vi "FPGA_Twosetup.vi"() -> ()   [LabVIEW 2015]
uses:
  <vilib>/rvi/Emulation/niFpgaGetClockAttributes.vi
  <vilib>/rvi/Emulation/niFpgaSctlEmulationGetInTimedLoop.vi
  <vilib>/rvi/Emulation/niFpgaEmulationReportErrorSimple.vi
  <vilib>/rvi/eio/common/nirviEmuTemplateMethod_errors.vi
  <vilib>/rvi/interface/RandomDataEmulation/niFpgaRandomDataHandleErrors.vi
  <vilib>/rvi/Emulation/niFpgaCriticalErrorInLSC.vi
  <vilib>/eio/EIONode/EIONode.xnode
  <vilib>/rvi/DataTransferAndStorage/Container/XNode/niFpgaContainer.xnode
  <vilib>/rvi/interface/RandomDataEmulation/nirviRandomDataFpgaReadWriteTemplate.vi
panel:
  in  "stop LED illumination 2":bool
  in  "Low Period (ticks) 2":u32=40000000
  in  "High Period (ticks) 2":u32=40000000
  in  "Apply 2":bool
  in  "Output Enable 2":bool
  in  "FPGA Stop 2":bool
  in  "Half-clock time 2":u32=10
  out "ConnectorA/DIO0 2":bool=TRUE
  out "Frame Count 2":i16=5
  in  "IRQ Bit (0-31) 2":u8
  in  "Wait Until IRQ Cleared? 2":bool
  out "Timed Out? 2":bool
  out "ConnectorA/AI0 2":u16=44020
  out "ConnectorA/DIO1 2":bool
  in  "double number of samples to take per frame 2":u16=1540
  in  "Half-clocks between frames 2":u16=1600
  in  "ConnectorA/AO0 2":u16
  in  "stop LED illumination":bool
  in  "Low Period (ticks)":u32=40000000
  in  "High Period (ticks)":u32=40000000
  in  "Apply":bool
  in  "Output Enable":bool
  in  "FPGA Stop":bool
  in  "Half-clock time":u32=10
  out "ConnectorB/DIO0":bool=TRUE
  out "Frame Count":i16=5
  in  "IRQ Bit (0-31)":u8
  in  "Wait Until IRQ Cleared?":bool
  out "Timed Out?":bool
  out "ConnectorB/AI0":u16=44020
  out "ConnectorB/DIO1":bool
  in  "double number of samples to take per frame":u16=1540
  in  "Half-clocks between frames":u16=1600
  in  "ConnectorB/AO0":u16
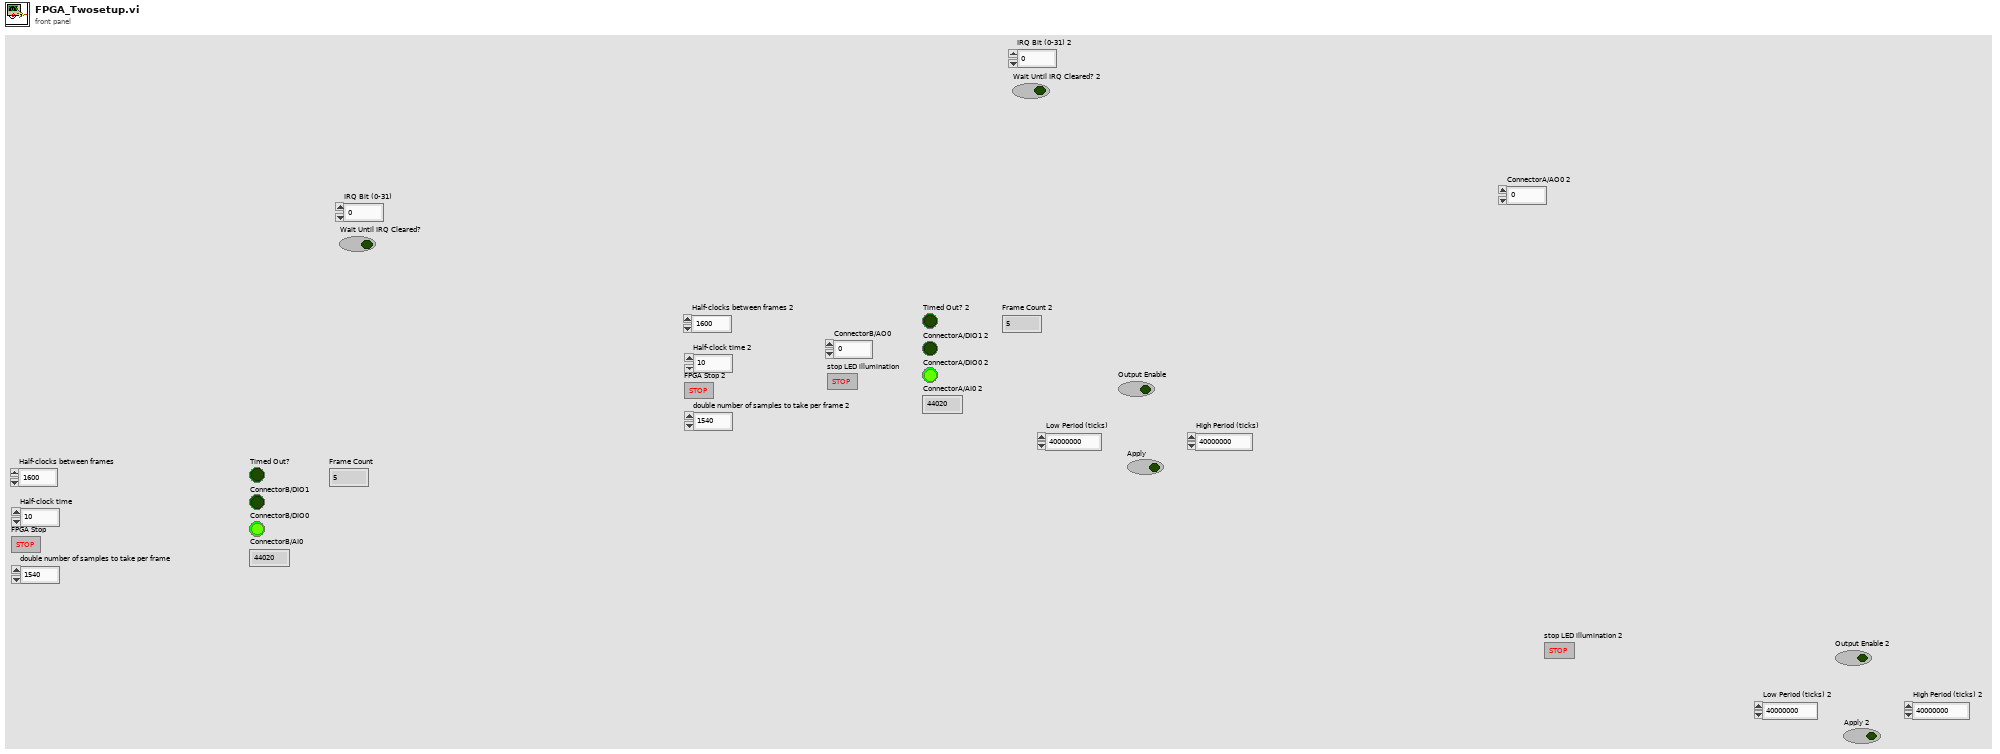
[diagram p1: front panel]
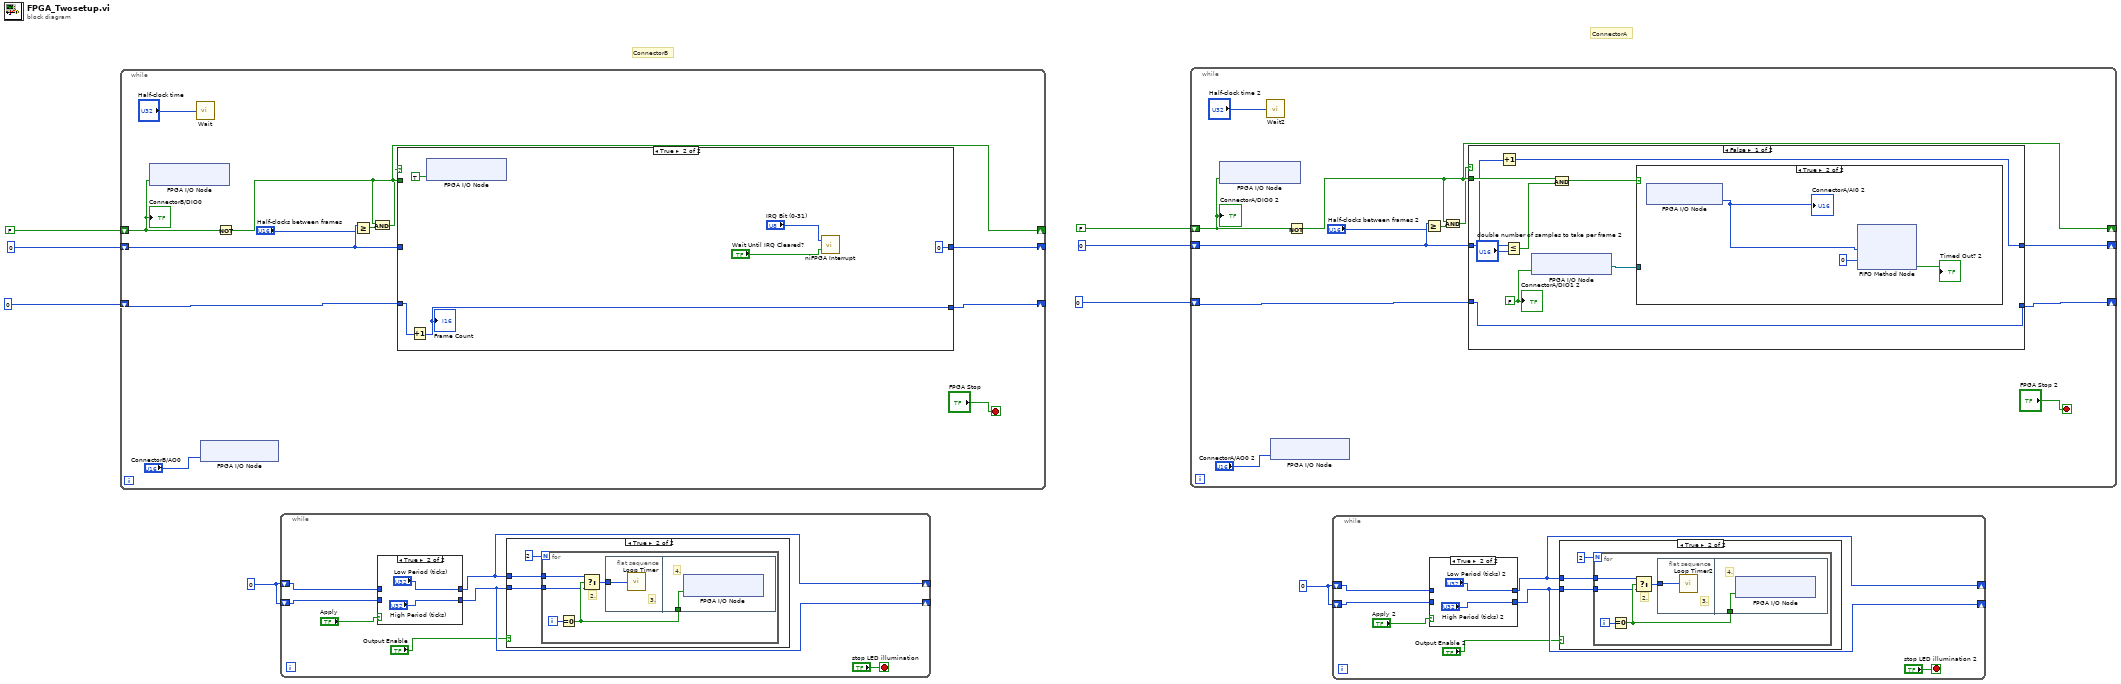
[diagram p0: block diagram]
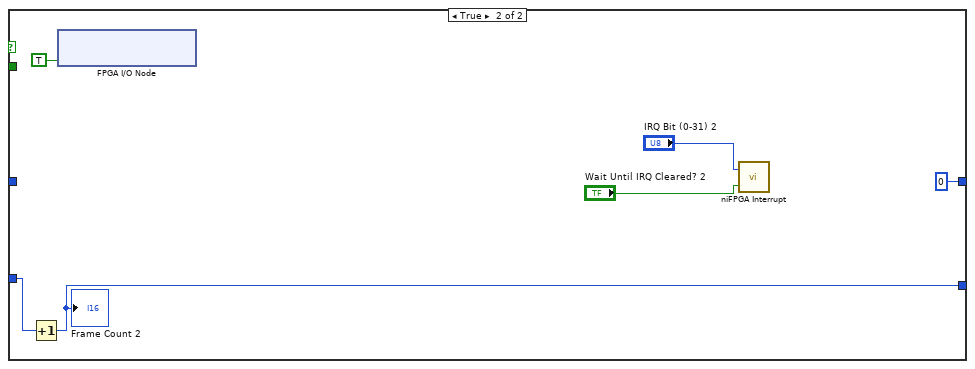
[diagram p5: hidden frame]
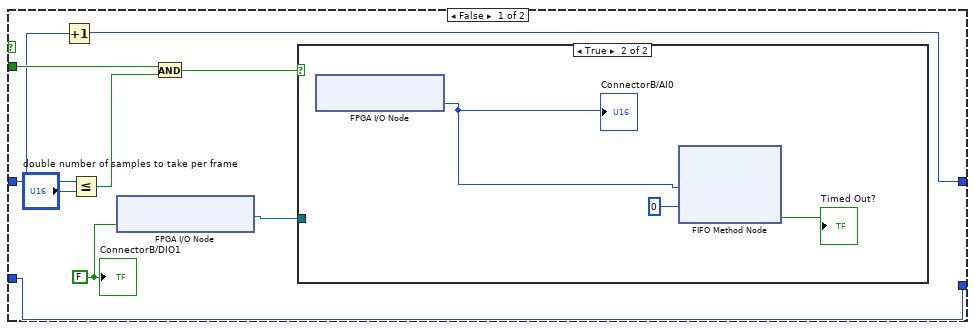
[diagram p8: hidden frame]
diagram:
  w1 = u32 0 ("High Period")
  w5 = u32 0 ("High Period")
  # "ConnectorA"
  # "ConnectorB"
  n1 = while {
    shift-right: [w19] -> _
    shift-left: FALSE ("ConnectorB/DIO0") -> [w20]
    shift-right: [w16] -> _
    shift-left: u16 0 -> [w18]
    shift-right: [w14] -> _
    shift-left: i16 0 -> [w15]
    stop <- "FPGA Stop" stop-if-true
    n2 = xnode "FPGA I/O Node"("ConnectorB/DIO0"=w20) -> ()  [unwired: 1 in, 1 out]
    n3 = call "Wait"("Count(uSec)"="Half-clock time") -> ()  [unwired: 1 out]
    n4 = xnode "FPGA I/O Node"("ConnectorB/AO0"="ConnectorB/AO0") -> ()  [unwired: 1 in, 1 out]
    n5 = Not(x=w20) -> (.not. x?=w19:bool)
    n6 = Greater Or Equal?(x=w18, y="Half-clocks between frames") -> (x >= y?=w12:bool)
    n7 = And(x=w19, y=w12) -> (x .and. y?=w10:bool)
    n8 = case shown="True" w10 {
      tunnel: w18 -> [w24 _]
      tunnel: [w22 u16 0] -> w16
      tunnel: w19 -> [w28 _]
      tunnel: w15 -> [w23 w36]
      tunnel: [w23 w35] -> w14
      frame False {
        w29 = FALSE ("ConnectorB/DIO1")
        n9 = Increment(x=w24) -> (x+1=w22:u16)
        n10 = Less Or Equal?(x=w24, y="double number of samples to take per frame") -> (x <= y?=w26:bool)
        n11 = xnode "FPGA I/O Node"("ConnectorB/DIO1"=w29) -> ("FPGA I/O Out"=w25:refnum<k21>)  [unwired: 1 in]
        n12 = And(x=w28, y=w26) -> (x .and. y?=w27:bool)
        n13 = case shown="True" w27 {
          tunnel: w25 -> [_ _]
          frame False {
          }
          frame True {
            n14 = xnode "FPGA I/O Node"() -> ("ConnectorB/AI0"=w32:u16)  [unwired: 1 in, 1 out]
            "ConnectorB/AI0" <- w32
            n15 = xnode ("FIFO Method Node")("Element"=w32, "Timeout"=0) -> ("Timed Out?"=→"Timed Out?":bool)  [unwired: 1 in, 1 out]
          }
        }
        "ConnectorB/DIO1" <- w29
      }
      frame True {
        n16 = Increment(x=w36) -> (x+1=w35:i16)
        "Frame Count" <- w35
        n17 = xnode "FPGA I/O Node"("ConnectorB/DIO1"=TRUE) -> ()  [unwired: 1 in, 1 out]
        n18 = call <vilib>:"niFPGA Interrupt.vi"("Wait Until Cleared (F)"="Wait Until IRQ Cleared?", "IRQ Number (0)"="IRQ Bit (0-31)") -> ()  [unwired: 1 in]
      }
    }
    "ConnectorB/DIO0" <- w20
  }
  n19 = while {
    shift-right: [w40] -> _
    shift-left: w5 -> [w44]
    shift-right: [w41] -> _
    shift-left: w5 -> [w43]
    stop <- "stop LED illumination" stop-if-true
    n20 = case shown="True" "Apply" {
      tunnel: [w57 "Low Period (ticks)"] -> w40
      tunnel: [w56 "High Period (ticks)"] -> w41
      tunnel: w44 -> [w57 _]
      tunnel: w43 -> [w56 _]
      frame False {
      }
      frame True {
      }
    }
    n21 = case shown="True" "Output Enable" {
      tunnel: w40 -> [_ w47]
      tunnel: w41 -> [_ w46]
      frame False {
      }
      frame True {
        n22 = for {
          N: 2 -> [_]
          tunnel: w47 -> [w50]
          tunnel: w46 -> [w49]
          i -> [w52]
          # "2."
          n23 = Equal To 0?(x=w52) -> (x = 0?=w51:bool)
          n24 = Select(t=w50, s=w51, f=w49) -> (s? t:f=w53:u32)
          n25 = flat-sequence {
            tunnel: w53 -> [w54]
            tunnel: w51 -> [w55]
            frame #0 {
              # "3."
              n26 = call "Loop Timer"("Count(Ticks)"=w54) -> ()  [unwired: 1 out]
            }
            frame #1 {
              # "4."
              n27 = xnode "FPGA I/O Node"("ConnectorB/DIO8"=w55) -> ()  [unwired: 1 in, 1 out]
            }
          }
        }
      }
    }
  }
  n28 = while {
    shift-right: [w70] -> _
    shift-left: FALSE ("ConnectorB/DIO0") -> [w71]
    shift-right: [w67] -> _
    shift-left: u16 0 -> [w69]
    shift-right: [w65] -> _
    shift-left: i16 0 -> [w66]
    stop <- "FPGA Stop 2" stop-if-true
    n29 = xnode "FPGA I/O Node"("ConnectorA/DIO0"=w71) -> ()  [unwired: 1 in, 1 out]
    n30 = call "Wait2"("Count(uSec)"="Half-clock time 2") -> ()  [unwired: 1 out]
    n31 = xnode "FPGA I/O Node"("ConnectorA/AO0"="ConnectorA/AO0 2") -> ()  [unwired: 1 in, 1 out]
    n32 = Not(x=w71) -> (.not. x?=w70:bool)
    n33 = Greater Or Equal?(x=w69, y="Half-clocks between frames 2") -> (x >= y?=w63:bool)
    n34 = And(x=w70, y=w63) -> (x .and. y?=w61:bool)
    n35 = case shown="False" w61 {
      tunnel: w69 -> [w75 _]
      tunnel: [w73 u16 0] -> w67
      tunnel: w70 -> [w79 _]
      tunnel: w66 -> [w74 w87]
      tunnel: [w74 w86] -> w65
      frame False {
        w80 = FALSE ("ConnectorB/DIO1")
        n36 = Increment(x=w75) -> (x+1=w73:u16)
        n37 = Less Or Equal?(x=w75, y="double number of samples to take per frame 2") -> (x <= y?=w77:bool)
        n38 = xnode "FPGA I/O Node"("ConnectorA/DIO1"=w80) -> ("FPGA I/O Out"=w76:refnum<k21>)  [unwired: 1 in]
        n39 = And(x=w79, y=w77) -> (x .and. y?=w78:bool)
        n40 = case shown="True" w78 {
          tunnel: w76 -> [_ _]
          frame False {
          }
          frame True {
            n41 = xnode "FPGA I/O Node"() -> ("ConnectorA/AI0"=w83:u16)  [unwired: 1 in, 1 out]
            "ConnectorA/AI0 2" <- w83
            n42 = xnode ("FIFO Method Node")("Element"=w83, "Timeout"=0) -> ("Timed Out?"=→"Timed Out? 2":bool)  [unwired: 1 in, 1 out]
          }
        }
        "ConnectorA/DIO1 2" <- w80
      }
      frame True {
        n43 = Increment(x=w87) -> (x+1=w86:i16)
        "Frame Count 2" <- w86
        n44 = xnode "FPGA I/O Node"("ConnectorA/DIO1"=TRUE ("ConnectorB/DIO1")) -> ()  [unwired: 1 in, 1 out]
        n45 = call <vilib>:"niFPGA Interrupt.vi"("Wait Until Cleared (F)"="Wait Until IRQ Cleared? 2", "IRQ Number (0)"="IRQ Bit (0-31) 2") -> ()  [unwired: 1 in]
      }
    }
    "ConnectorA/DIO0 2" <- w71
  }
  n46 = while {
    shift-right: [w91] -> _
    shift-left: w1 -> [w95]
    shift-right: [w92] -> _
    shift-left: w1 -> [w94]
    stop <- "stop LED illumination 2" stop-if-true
    n47 = case shown="True" "Apply 2" {
      tunnel: [w108 "Low Period (ticks) 2"] -> w91
      tunnel: [w107 "High Period (ticks) 2"] -> w92
      tunnel: w95 -> [w108 _]
      tunnel: w94 -> [w107 _]
      frame False {
      }
      frame True {
      }
    }
    n48 = case shown="True" "Output Enable 2" {
      tunnel: w91 -> [_ w98]
      tunnel: w92 -> [_ w97]
      frame False {
      }
      frame True {
        n49 = for {
          N: 2 -> [_]
          tunnel: w98 -> [w101]
          tunnel: w97 -> [w100]
          i -> [w103]
          # "2."
          n50 = Equal To 0?(x=w103) -> (x = 0?=w102:bool)
          n51 = Select(t=w101, s=w102, f=w100) -> (s? t:f=w104:u32)
          n52 = flat-sequence {
            tunnel: w104 -> [w105]
            tunnel: w102 -> [w106]
            frame #0 {
              # "3."
              n53 = call "Loop Timer2"("Count(Ticks)"=w105) -> ()  [unwired: 1 out]
            }
            frame #1 {
              # "4."
              n54 = xnode "FPGA I/O Node"("ConnectorA/DIO8"=w106) -> ()  [unwired: 1 in, 1 out]
            }
          }
        }
      }
    }
  }
